vi "niFPGA Discrete Normalized Integrator_m.vi"   [LabVIEW 2017]
doc: "Integrates a discrete input signal using forward Euler integration. The VI assumes that the integration interval (dt) is normalized to 1. The data type you wire to <B>input</B> determines <B>output</B> data type, where output word length is equal to input word length + 16 bits."
uses:
  <vilib>/rvi/Analysis/common/FxpNativeNode/niFpgaFxpNative.xnode
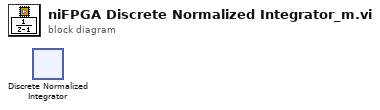
[diagram p0: block diagram]
diagram:
  n1 = xnode ("Discrete Normalized Integrator")() -> ()  [unwired: 3 in, 1 out]
